vi "External Sensor Sensitivities DAO.vi"(7 "refnum":T1, 8 "error in (no error)":errorcluster, 10 "Sensitivities In":dbl[](array[numeric]), 11 "Persistent DAO Actions":T2) -> (0 "error out":errorcluster, 2 "Sensitivities Out":dbl[](array[numeric]), 4 "refnum out":T1)   [LabVIEW 2013]
uses:
  Metadata/Persistant DAO Actions.ctl
  <vilib>/Utility/config.llb/Config Data RefNum.ctl
  <vilib>/Utility/config.llb/NI_LVConfig.lvlib
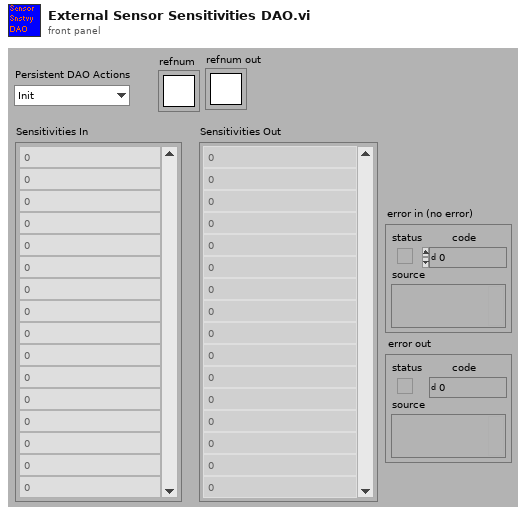
[diagram p1: front panel]
types:
  T1 = typedef "NI_LVConfig.lvlib/Config Data RefNum.ctl" = refnum<k1>
  T2 = typedef "Persistant DAO Actions.ctl" = enum16{"Init", "Get", "Set", "Load", "Save"}
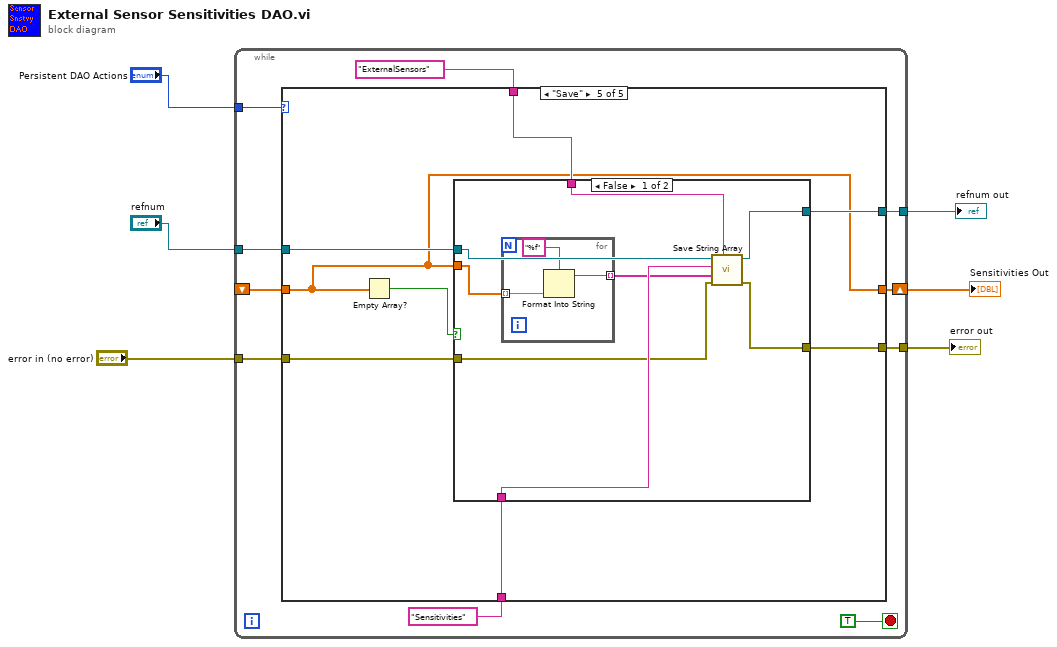
[diagram p0: block diagram]
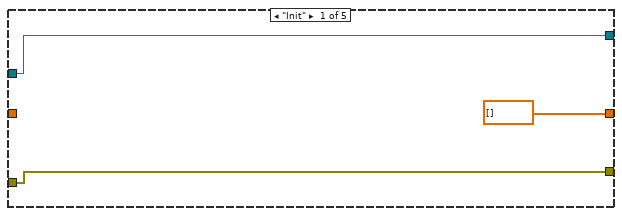
[diagram p2: hidden frame]
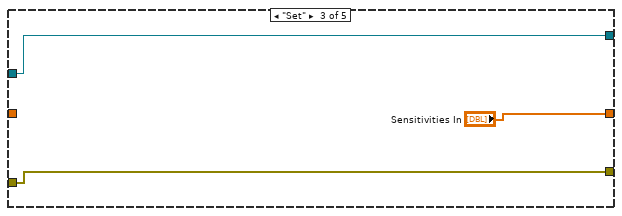
[diagram p4: hidden frame]
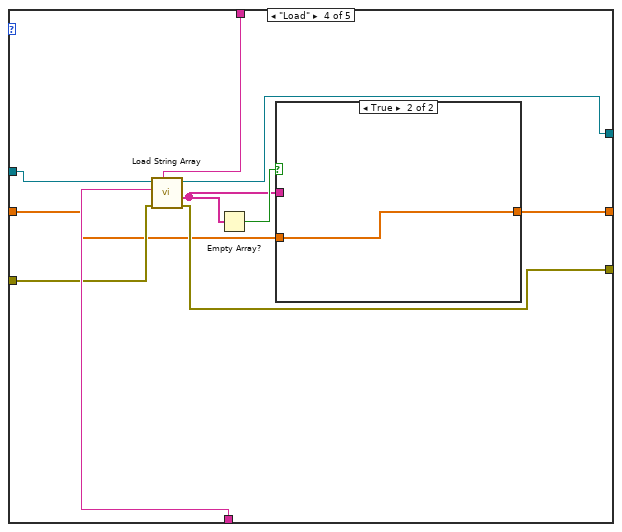
[diagram p5: hidden frame]
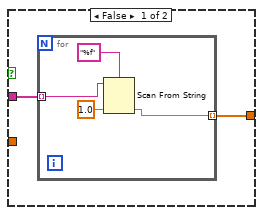
[diagram p6: hidden frame]
diagram:
  n1 = while {
    tunnel: "Persistent DAO Actions" -> [w15]
    shift-right: [w14] -> w5
    shift-left: _ -> [w13]
    tunnel: "refnum" -> [w12]
    tunnel: "error in (no error)" -> [w9]
    tunnel: [w8] -> w2
    tunnel: [w7] -> w1
    stop <- TRUE stop-if-true
    n2 = case shown="\"Save\"" w15 {
      tunnel: [dbl[] [] ("Sensitivities In") w22 "Sensitivities In" w27 w43] -> w14
      tunnel: w13 -> [_ w22 _ w26 w43]
      tunnel: w12 -> [w19 w21 w24 w33 w49]
      tunnel: "Sensitivities" -> [_ _ _ w35 w48]
      tunnel: "ExternalSensors" -> [_ _ _ w34 w47]
      tunnel: w9 -> [w18 w20 w23 w31 w46]
      tunnel: [w19 w21 w24 w32 w45] -> w8
      tunnel: [w18 w20 w23 w30 w44] -> w7
      frame "Init" {
      }
      frame "Get" {
      }
      frame "Set" {
      }
      frame "Load" {
        n3 = call "Load String Array.vi"("section"=w34, "error in (no error)"=w31, "key"=w35, "refnum"=w33) -> ("error out"=w30:errorcluster, "String Array Out"=w28:string[], "refnum out"=w32:T1)  [unwired: 5 out]
        n4 = Empty Array?(array=w28) -> (empty?=w29:bool)
        n5 = case shown="True" w29 {
          tunnel: w28 -> [w37 _]
          tunnel: [w36 w42] -> w27
          tunnel: w26 -> [_ w42]
          frame False {
            n6 = for {
              tunnel: w37 -> [w41] mode=indexing
              tunnel: [w38] -> w36 mode=indexing
              n7 = Scan From String(format string="%f", input string=w41, default 1=1.0 ("default value 1")) -> (output 1=w38:dbl)  [unwired: 2 in, 3 out]
            }
          }
          frame True {
          }
        }
      }
      frame "Save" {
        n8 = Empty Array?(array=w43) -> (empty?=w50:bool)
        n9 = case shown="False" w50 {
          tunnel: w43 -> [w52 _]
          tunnel: w49 -> [w58 w63]
          tunnel: w48 -> [w57 _]
          tunnel: w47 -> [w56 _]
          tunnel: w46 -> [w55 w62]
          tunnel: [w54 w63] -> w45
          tunnel: [w53 w62] -> w44
          frame False {
            n10 = for {
              tunnel: w52 -> [w61] mode=indexing
              tunnel: [w60] -> w51 mode=indexing
              n11 = Format Into String(format string="%f", w61) -> (resulting string=w60:string)  [unwired: 2 in, 1 out]
            }
            n12 = call "Save String Array.vi"("section"=w56, "error in (no error)"=w55, "String Array In"=w51, "key"=w57, "refnum"=w58) -> ("error out"=w53:errorcluster, "refnum out"=w54:T1)  [unwired: 5 out]
          }
          frame True {
          }
        }
      }
    }
  }
  "Sensitivities Out" <- w5
  "refnum out" <- w2
  "error out" <- w1
